vi "_FPGA_wfmFXPtoU14.vi"(1 "wfmFXP":fxp<+/-,16,14>) -> (0 "U14":fxp<+,14,14>)   [LabVIEW 2018]
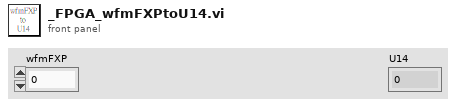
[diagram p1: front panel]
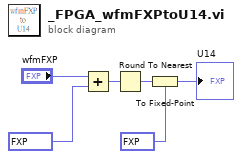
[diagram p0: block diagram]
diagram:
  n1 = Add(x="wfmFXP", y=fxp<+/-,16,14> 8191.5) -> (x+y=w3:fxp<+/-,17,15>)
  n2 = Round To Nearest(number=w3) -> (nearest integer value=w5:fxp<+/-,16,16>)
  n3 = To Fixed-Point(fixed-point type=fxp<+,14,14> 8192.0, number=w5) -> (fixed-point=→"U14":fxp<+,14,14>)
